vi "StimFile-Read Reference.vi"(0 "Wave File":path, 7 "refUnits":string="refSPL", 9 "Destination":string, 11 "error in (no error)":errorcluster) -> (4 "Reference (dB)":dbl, 8 "Units":string, 15 "error out":errorcluster)   [LabVIEW 2020]
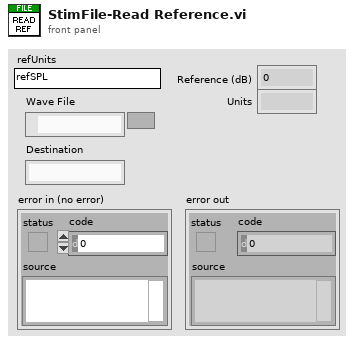
[diagram p1: front panel]
types:
  T1 = typedef "Wave-EPL Chunk Variable.ctl" = cluster{"Name":string, "Value":dbl}
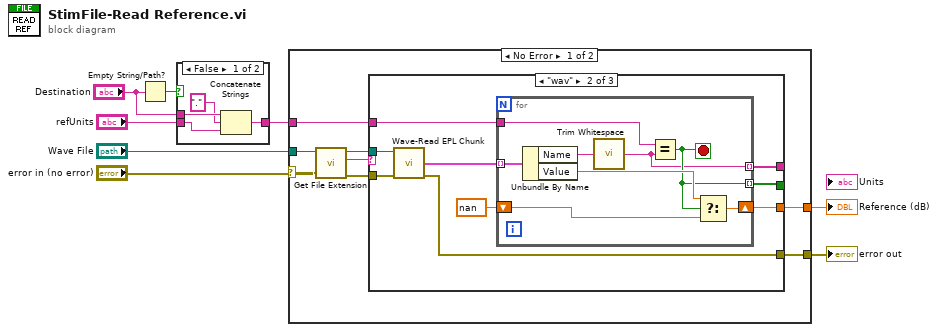
[diagram p0: block diagram]
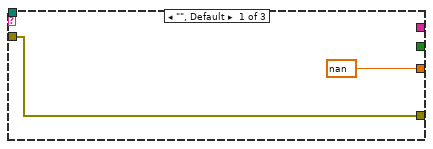
[diagram p3: hidden frame]
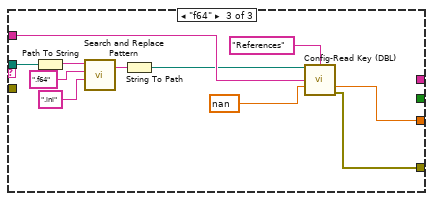
[diagram p4: hidden frame]
diagram:
  n1 = Empty String/Path?(string/path="Destination") -> (empty?=w4:bool)
  n2 = case shown="False" w4 {
    tunnel: [w12 w13] -> w3
    tunnel: "refUnits" -> [w10 w13]
    tunnel: "Destination" -> [w11 _]
    frame False {
      n3 = Concatenate Strings(w11, "." ("string"), w10) -> (w12:string)
    }
    frame True {
    }
  }
  n4 = case shown="No Error" "error in (no error)" {
    selector: "error in (no error)" -> [w15 w52]
    tunnel: [w21 w52] -> w7
    tunnel: "Wave File" -> [w16 _]
    tunnel: [w20 _] -> w5
    tunnel: w3 -> [w19 _]
    frame No Error {
      n5 = call <vilib>:"Get File Extension.vi"("error in (no error)"=w15, "file"=w16) -> ("error out"=w18:errorcluster, "lowercase file extension"=w14:string, "dup file"=w17:path)  [unwired: 5 in, 2 out]
      n6 = case shown="\"wav\"" w14 {
        tunnel: [w23 w30 w47] -> w21
        tunnel: [nan w29 w49] -> w20
        tunnel: w19 -> [_ w28 w50]
        tunnel: w18 -> [w23 w27 _]
        tunnel: w17 -> [_ w26 w46]
        tunnel: [_ w25 _] -> _
        tunnel: [_ w24 _] -> _
        frame "", Default {
        }
        frame "wav" {
          n7 = call "Wave-Read EPL Chunk.vi"("Wave File"=w26, "error in (no error)"=w27) -> ("EPL Variables"=w32:T1[], "error out"=w30:errorcluster)  [unwired: 12 in]
          n8 = for {
            tunnel: w32 -> [w40] mode=indexing
            shift-right: [w37] -> w29
            shift-left: nan -> [w38]
            tunnel: w28 -> [w36]
            tunnel: [w33] -> w25 mode=indexing
            tunnel: [w34] -> w24 mode=indexing
            stop <- w34 stop-if-true
            n9 = Unbundle By Name(w40) -> ("Name"=w35:string, "Value"=w39:dbl)
            n10 = call <vilib>:"Trim Whitespace.vi"("string"=w35) -> ("trimmed string"=w33:string)  [unwired: 1 in]
            n11 = Equal?(x=w36, y=w33) -> (x = y?=w34:bool)
            n12 = Select(t=w39, s=w34, f=w38) -> (s? t:f=w37:dbl)
          }
        }
        frame "f64" {
          n13 = Path To String(path=w46) -> (string=w45:string)
          n14 = call <vilib>:"Search and Replace Pattern.vi"("string"=w45, "regular expression (\"\")"=".f64" ("regular expression (\"\")"), "replace string (\"\")"=".ini" ("replace string (\"\")")) -> ("result string"=w42:string)  [unwired: 2 in, 1 out]
          n15 = String To Path(string=w42) -> (path=w41:path)
          n16 = call "Config-Read Key (DBL).vi"("configuration file path"=w41, "section"="References", "key"=w50, "default"=nan) -> ("value"=w49:dbl, "error out"=w47:errorcluster)  [unwired: 8 in, 2 out]
        }
      }
    }
    frame Error {
    }
  }
  "error out" <- w7
  "Reference (dB)" <- w5
